vi "fgv_PotentialField_set-val.vi"(7 "cmd":T2, 11 "set-val":T3={"start pt"={"x"=0.0, "y"=10.0}, "goal pt"={"x"=30.0, "y"=30.0}, "grid size"=0.5, "robot radius"=5.0, "obstacles"=[{"x"=15, "y"=25}, {"x"=5, "y"=15}, {"x"=20, "y"=26}, {"x"=25, "y"=25}]}) -> (3 "set-val out":T1={"start pt"={"x"=0.0, "y"=10.0}, "goal pt"={"x"=30.0, "y"=30.0}, "grid size"=0.5, "robot radius"=5.0, "obstacles"=[{"x"=15.0, "y"=25.0}, {"x"=5.0, "y"=15.0}, {"x"=20.0, "y"=26.0}, {"x"=25.0, "y"=25.0}]})   [LabVIEW 2019]
uses:
  Ctrl/cmd_common.ctl
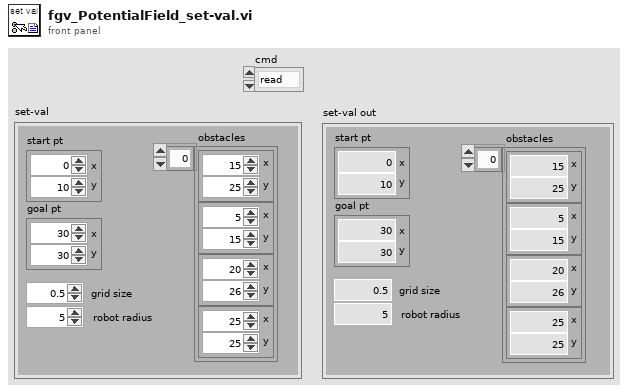
[diagram p1: front panel]
types:
  T1 = cluster{"start pt":cluster{"x":dbl, "y":dbl}, "goal pt":cluster{"x":dbl, "y":dbl}, "grid size":dbl, "robot radius":dbl, "obstacles":cluster{"x":dbl, "y":dbl}[]}
  T2 = typedef "cmd_common.ctl" = enum16{"read", "write"}
  T3 = cluster{"start pt":cluster{"x":dbl, "y":dbl}, "goal pt":cluster{"x":dbl, "y":dbl}, "grid size":dbl, "robot radius":dbl, "obstacles":cluster{"x":i32, "y":i32}[]}
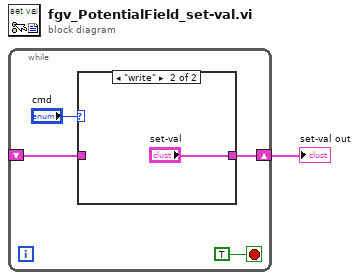
[diagram p0: block diagram]
diagram:
  n1 = while {
    shift-right: [w3] -> w1
    shift-left: _ -> [w2]
    stop <- TRUE stop-if-true
    n2 = case shown="\"write\"" "cmd" {
      tunnel: [w6 "set-val"] -> w3
      tunnel: w2 -> [w6 _]
      frame "read", Default {
      }
      frame "write" {
      }
    }
  }
  "set-val out" <- w1
